vi "12-1-a.vi"(9 "route in":string[](array[string]), 10 "Numeric":i32, 11 "Array":T1(array[cluster])) -> (1 "Route out":string[][](array[string]))   [LabVIEW 2019, in "12.lvlib"]
uses:
  12.lvlib
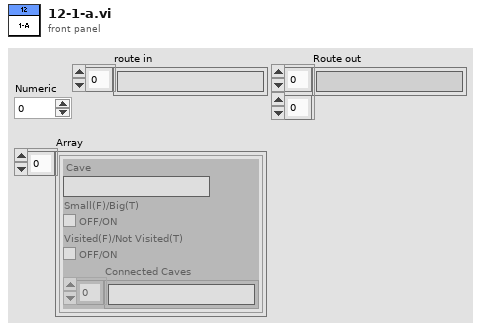
[diagram p1: front panel]
types:
  T1 = cluster{"Cave":string, "Small(F)/Big(T)":bool, "Visited(F)/Not Visited(T)":bool, "Connected Caves":string[]}[]
  T2 = cluster{"Cave":string, "Small(F)/Big(T)":bool, "Visited(F)/Not Visited(T)":bool, "Connected Caves":string[]}
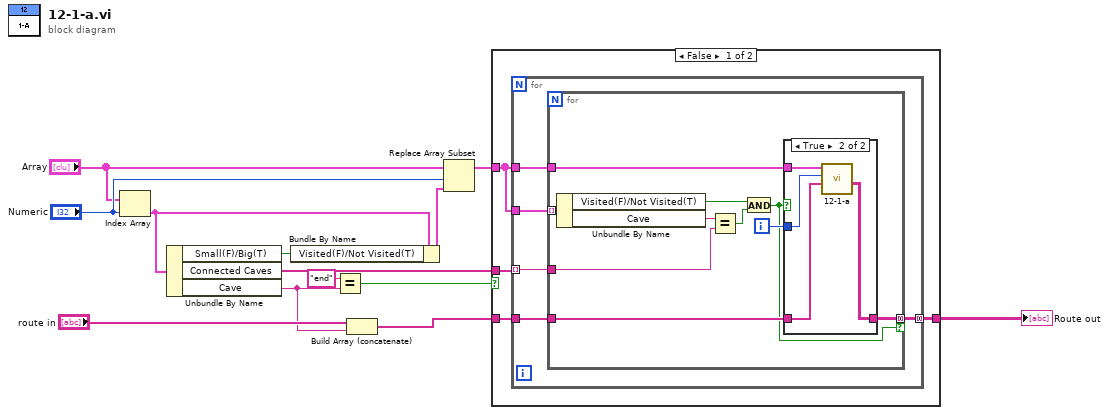
[diagram p0: block diagram]
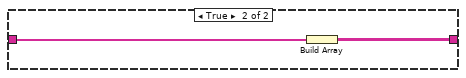
[diagram p3: hidden frame]
diagram:
  n1 = Index Array(array="Array", index="Numeric") -> (element=w11:T2)
  n2 = Unbundle By Name(w11) -> ("Small(F)/Big(T)"=w9:bool, "Connected Caves"=w12:string[], "Cave"=w1:string)
  n3 = Bundle By Name(cluster=w11, "Visited(F)/Not Visited(T)"=w9) -> (w13:T2)
  n4 = Equal?(x="end" ("y"), y=w1) -> (x = y?=w8:bool)
  n5 = Build Array (concatenate)("route in", w1) -> (w4:string[])
  n6 = Replace Array Subset(array="Array", new element=w13, index="Numeric") -> (w10:T1)
  n7 = case shown="False" w8 {
    tunnel: w12 -> [w17 _]
    tunnel: w10 -> [w16 _]
    tunnel: w4 -> [w15 w38]
    tunnel: [w14 w37] -> w2
    frame False {
      n8 = for {
        tunnel: w16 -> [w21]
        tunnel: w17 -> [w22] mode=indexing
        tunnel: w16 -> [w20]
        tunnel: w15 -> [w19]
        tunnel: [w18] -> w14 mode=concatenating
        n9 = for {
          tunnel: w22 -> [w31]
          tunnel: w21 -> [w28] mode=indexing
          tunnel: w20 -> [w27]
          tunnel: w19 -> [w26]
          tunnel: [w24] -> w18 mode=concatenating if=w23
          i -> [w25]
          n10 = Unbundle By Name(w28) -> ("Visited(F)/Not Visited(T)"=w29:bool, "Cave"=w32:string)
          n11 = Equal?(x=w32, y=w31) -> (x = y?=w30:bool)
          n12 = And(x=w29, y=w30) -> (x .and. y?=w23:bool)
          n13 = case shown="True" w23 {
            tunnel: w27 -> [_ w36]
            tunnel: w25 -> [_ w35]
            tunnel: w26 -> [_ w34]
            tunnel: [_ w33] -> w24
            frame False {
            }
            frame True {
              n14 = call "12-1-a.vi"("route in"=w34, "Numeric"=w35, "Array"=w36) -> ("Route out"=w33:string[][])  [unwired: 8 in]
            }
          }
        }
      }
    }
    frame True {
      n15 = Build Array(w38) -> (w37:string[][])
    }
  }
  "Route out" <- w2
